vi "Set AP Sx Ref Curve Val.vi"(0 "asicHandle":i32, 1 "rightY":dbl, 2 "upperLimit":dbl, 5 "leftX":dbl, 7 "leftY":dbl, 9 "rightX":dbl, 11 "error in (no error)":errorcluster caption="错误输入（无错误）", 12 "lowerLimit":dbl, 13 "yScale":dbl) -> (4 "function return":i32, 15 "error out":errorcluster caption="错误输出")   [LabVIEW 2018]
doc: "extern int __stdcall SetAPSxRefCurveVal (int asicHandle, IN double leftX, IN double leftY, IN double rightX, IN double rightY, IN double lowerLimit, IN double upperLimit, IN double yScale);"
uses:
  APSx.dll/APSx.dll
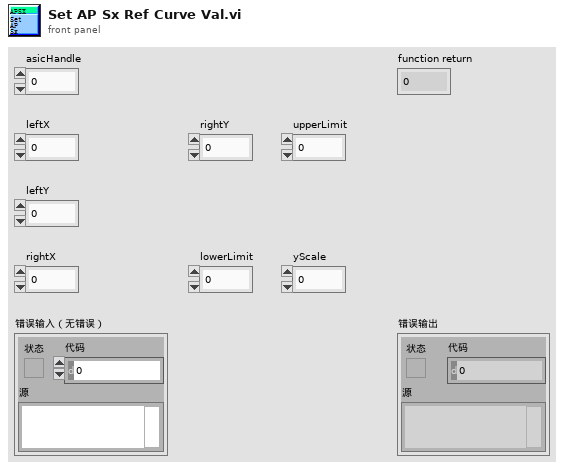
[diagram p1: front panel]
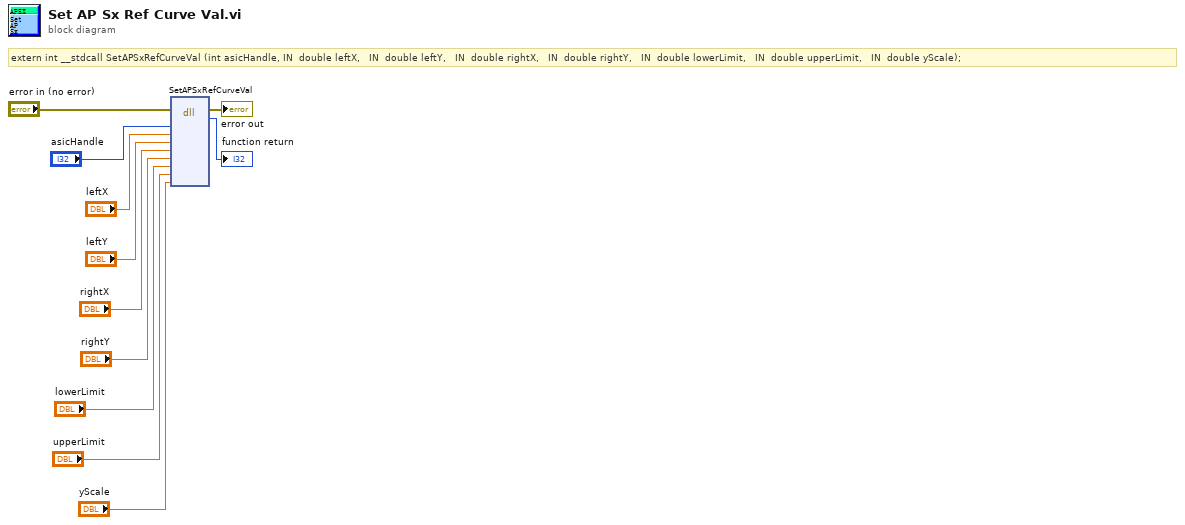
[diagram p0: block diagram]
diagram:
  # "extern int __stdcall SetAPSxRefCurveVal (int asicHandle, IN  double leftX,   IN  double leftY,   IN  double rightX,   IN  double rightY,   IN  double lowerLimit,   IN  double upperLimit,   IN  double yScale);"
  n1 = dll-call lib="PTH2[abs D项目Feng恒隆项目Labview传感器对中台SourcesAPSx.dllAPSx.*" fn="SetAPSxRefCurveVal"(error in="error in (no error)", "asicHandle"="asicHandle", "leftX"="leftX", "leftY"="leftY", "rightX"="rightX", "rightY"="rightY", "lowerLimit"="lowerLimit", "upperLimit"="upperLimit", "yScale"="yScale") -> (error out=→"error out":errorcluster, →"function return":i32)  [unwired: 10 in, 1 out]
